vi "x2dotTOx2.vi"(10 "x2dot":dbl, 11 "Array: x2dot":dbl[](array[numeric])) -> (2 "Array: x2dot":dbl[](array[numeric]), 3 "x2":dbl)   [LabVIEW 2013]
uses:
  <vilib>/Analysis/2dsp.llb/Integral Method.ctl
  <vilib>/Analysis/NI_AALPro.lvlib
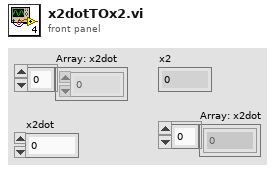
[diagram p1: front panel]
types:
  T1 = typedef "NI_AALPro.lvlib/Integral Method.ctl" = i32
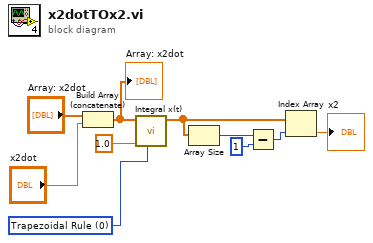
[diagram p0: block diagram]
diagram:
  w3 = T1 0 items=["Trapezoidal Rule", "Simpson's Rule", "Simpson's 3/8 Rule", "Bode Rule"] ("integration method")
  n1 = Build Array (concatenate)("Array: x2dot", "x2dot") -> (w8:dbl[])
  "Array: x2dot" <- w8
  n2 = call <vilib>:"Integral x(t).vi"("integration method"=w3, "dt"=1.0, "X"=w8) -> ("Integral X"=w4:dbl[])  [unwired: 7 in, 1 out]
  n3 = Array Size(array=w4) -> (size(s)=w5:i32)
  n4 = Subtract(x=w5, y=1) -> (x-y=w7:i32)
  n5 = Index Array(array=w4, index=w7) -> (element=→"x2":dbl)
